vi "Stop Pattern.vi"(8 "error in (no error)":errorcluster, 9 "Timeout":i32, 11 "CS++PPG in":refnum<class "CS++PPG.lvclass">) -> (0 "error out":errorcluster, 3 "CS++PPG out":refnum<class "CS++PPG.lvclass">)   [LabVIEW 2015, in "CS++PPG.lvlib" / "CS++PPG.lvclass"]
doc: "This VI stops the execution of the pattern."
uses:
  CS++PPG.lvclass
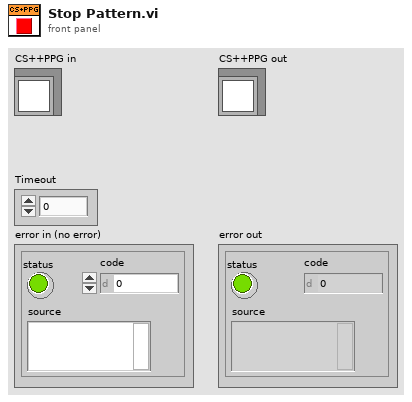
[diagram p1: front panel]
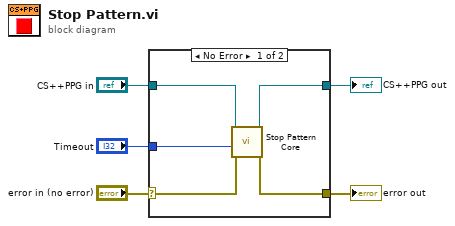
[diagram p0: block diagram]
diagram:
  n1 = case shown="No Error" "error in (no error)" {
    selector: "error in (no error)" -> [w9 w12]
    tunnel: [w8 w12] -> w4
    tunnel: [w7 w11] -> w2
    tunnel: "CS++PPG in" -> [w10 w11]
    tunnel: "Timeout" -> [w6 _]
    frame No Error {
      n2 = call-dynamic "Stop Pattern Core.vi"("error in (no error)"=w9, "Timeout"=w6, "CS++PPG in"=w10) -> ("error out"=w8:errorcluster, "CS++PPG out"=w7:refnum<class "CS++PPG.lvclass">)  [unwired: 7 in]
    }
    frame Error {
    }
  }
  "error out" <- w4
  "CS++PPG out" <- w2
